vi "Write test data to file polaris.vi"(0 "imei":string="ImeiImeiImeiIme", 1 "Meid":string="MediMeidMeidMe", 4 "SIM ID":string="SimSimSimSimSimSimID", 5 "Mac":string="MacMacMacMac", 7 "phone":string="ImeiImeiImeiIme", 9 "Serial Number":string="MediMeidMeidMe", 11 "error in (no error)":errorcluster, 14 "Style":string="100060") -> (10 "PassFail":string="Fail", 15 "error out":errorcluster)   [LabVIEW 2013]
uses:
  Test Globals/Global 1.vi
  Main Support/Global 2.vi
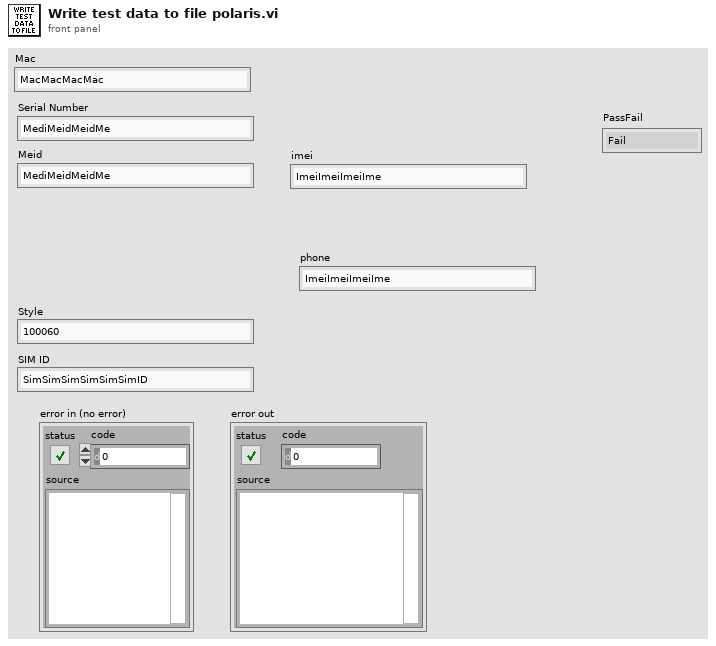
[diagram p1: front panel]
types:
  T1 = enum16{"Query", "Insert", "Select", "Dump Recs", "Get Rec Count", "Get Col Names", "Insert all fields", "Find", "Get last test result", "Get work order qty", "Set work order qty", "Save test report", "Get test report", "Execute query no data", "Select count", "Query and return row 0 col 0"}
  T2 = enum16{"get next serial available and assign", "change status to available", "assign a given serial number"}
  T3 = enum16{"get next serial available and assign", "change status to available"}
  T4 = cluster{"Test folder":string, "Top level":string, "Main":string, "Test report":string, "Work order qty":string, "Work order meid":string, "Work order imei":string, "Master meid imei list":string, "Master test data":string, "ZPL label info":string, "Pictures":string, "Setup info":string, "Work order":string, "Tests folder":string, "Tests steps folder":string, "Config folder":string, "Verizon Upload file":string, "Job data file":string, "Station globals":string, "Post test info":string}
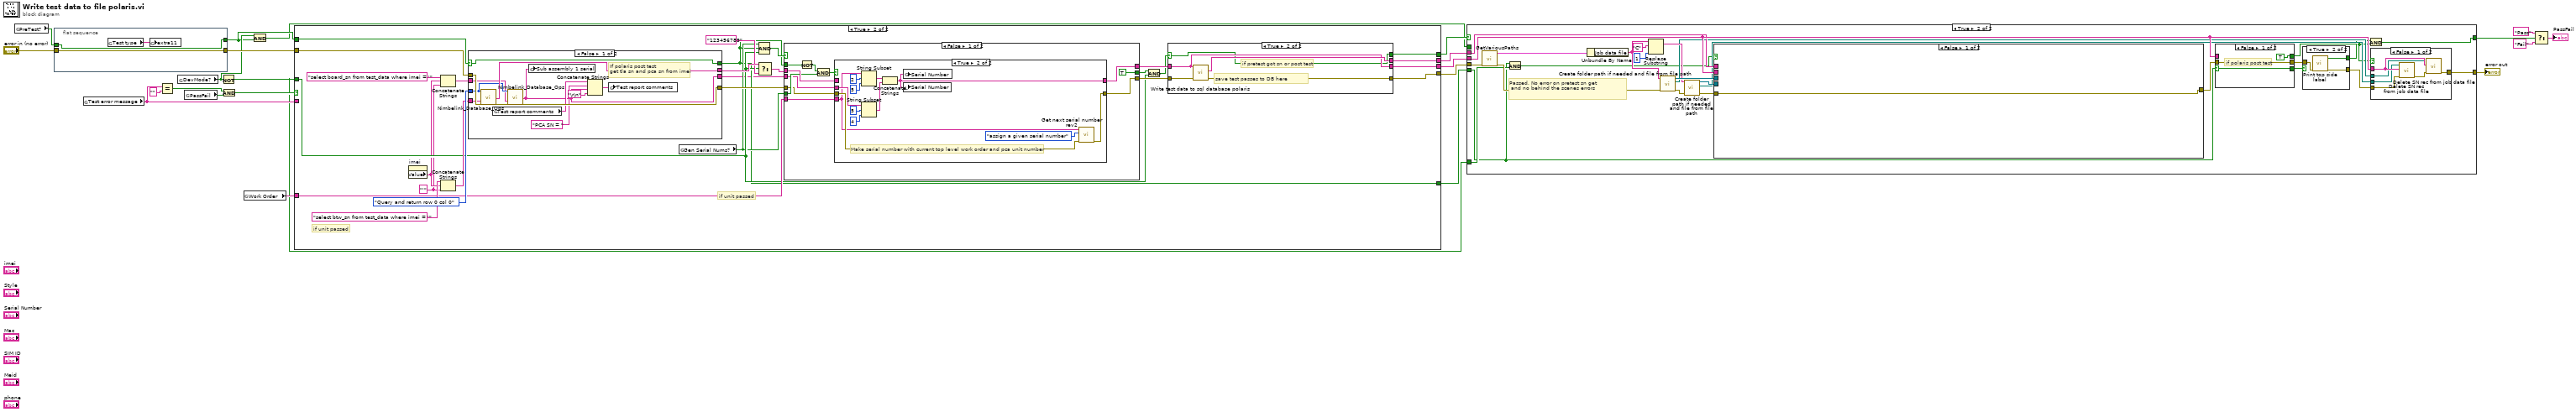
[diagram p0: block diagram]
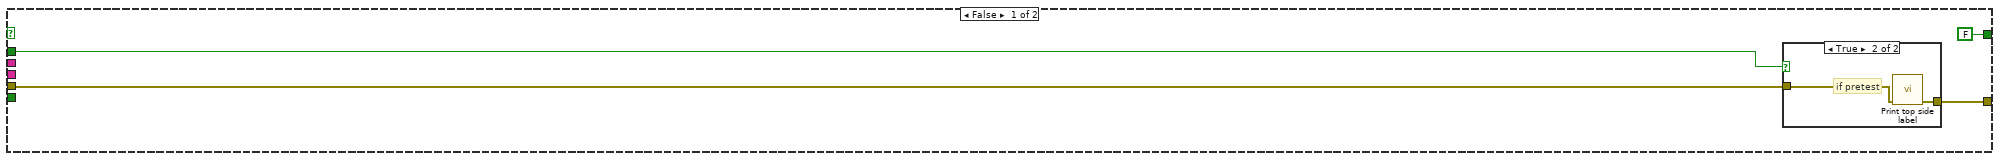
[diagram p2: hidden frame]
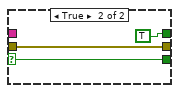
[diagram p4: hidden frame]
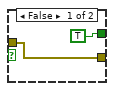
[diagram p5: hidden frame]
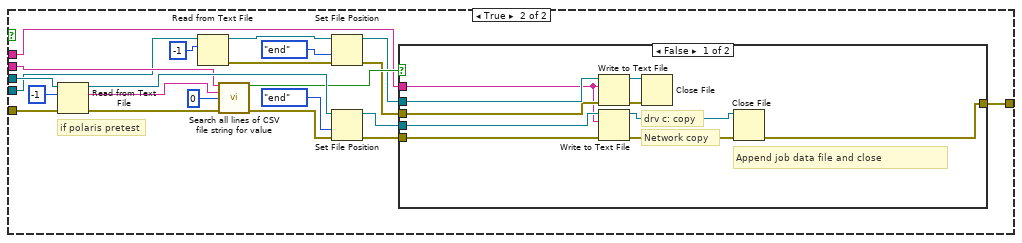
[diagram p7: hidden frame]
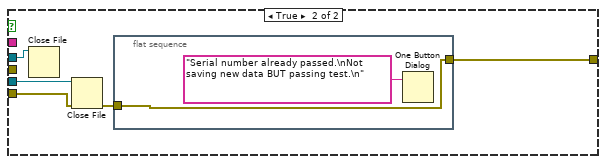
[diagram p8: hidden frame]
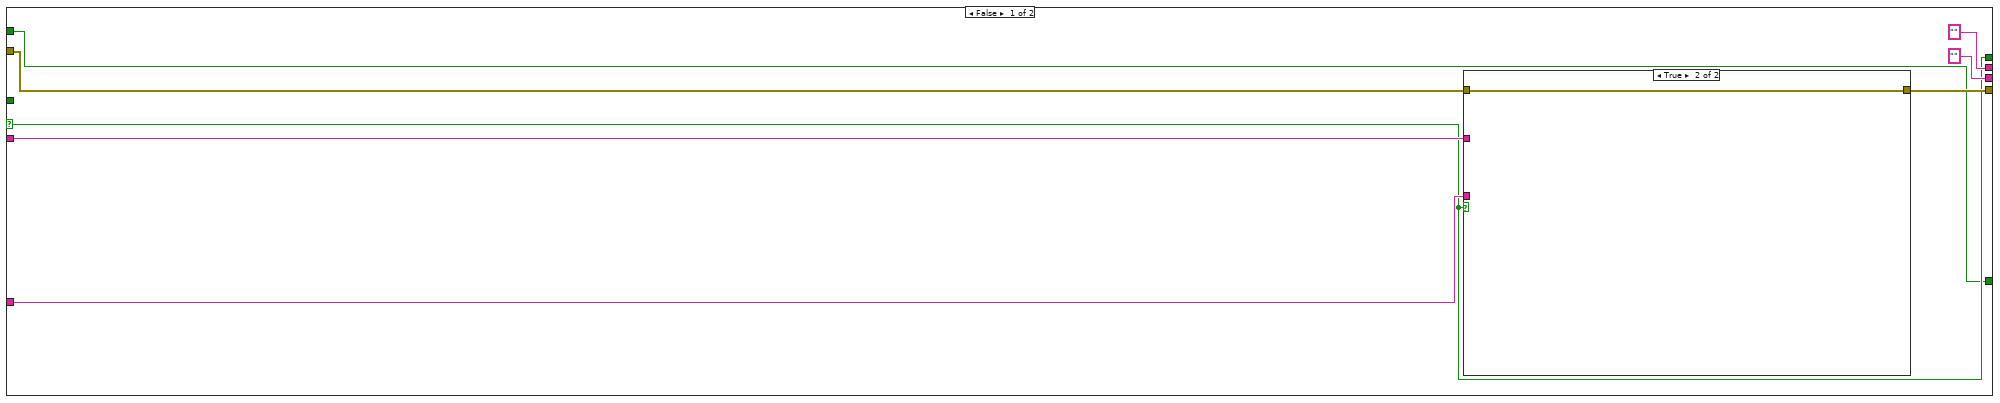
[diagram p9: hidden frame]
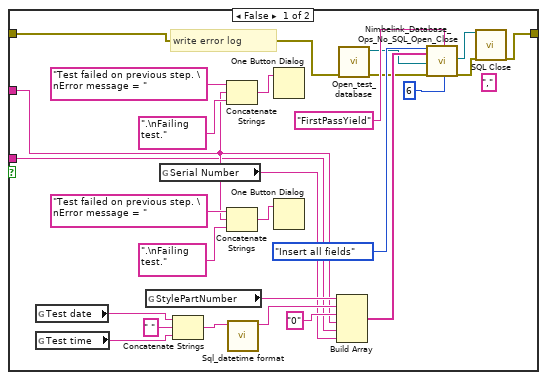
[diagram p10: hidden frame]
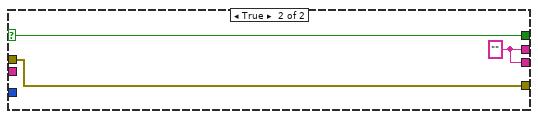
[diagram p11: hidden frame]
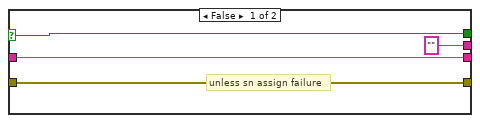
[diagram p12: hidden frame]
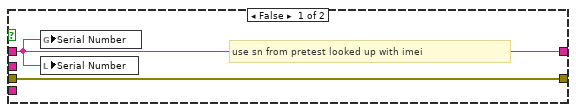
[diagram p13: hidden frame]
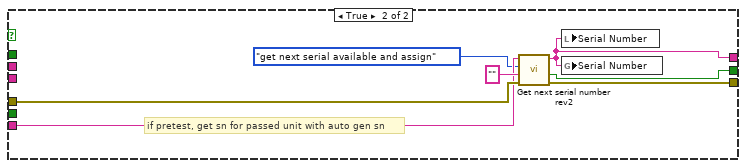
[diagram p14: hidden frame]
diagram:
  n1 = global read "Global 1.vi" "PreTest?"() -> (w7:bool)
  n2 = flat-sequence {
    tunnel: w7 -> [w25]
    tunnel: [w26] -> w9
    tunnel: "error in (no error)" -> [w26]
    tunnel: [w25] -> w2
    frame #0 {
      n3 = global read "Global 1.vi" "Test type"() -> (w24:string)
      n4 = global write "Global 1.vi" "extra11"(w24) -> ()
    }
  }
  n5 = global read "Global 1.vi" "Test error message"() -> (w14:string)
  n6 = Equal?(x=w14, y="") -> (x = y?=w18:bool)
  n7 = global read "Global 1.vi" "DevMode?"() -> (w3:bool)
  n8 = global read "Global 2.vi" "PassFail"() -> (w17:bool)
  n9 = Not(x=w3) -> (.not. x?=w4:bool)
  n10 = And(x=w18, y=w17) -> (x .and. y?=w15:bool)
  n11 = global read "Global 2.vi" "Work Order"() -> (w13:string)
  n12 = And(x=w3, y=w2) -> (x .and. y?=w1:bool)
  n13 = case shown="True" w15 {
    selector: w15 -> [w28 _]
    tunnel: [w30 w85] -> w12
    tunnel: w9 -> [w31 w83]
    tunnel: [w28 w84] -> w5
    tunnel: w14 -> [w34 _]
    tunnel: ["" ("Serial number out") w87] -> w11
    tunnel: ["" ("Test rec csv line") w86] -> w10
    tunnel: w13 -> [w29 w77]
    tunnel: w2 -> [w27 w64]
    tunnel: [w27 w66] -> w6
    tunnel: w4 -> [_ w68]
    frame False {
      n14 = case shown="True" w28 {
        tunnel: w34 -> [w38 _]
        tunnel: w31 -> [w39 w61]
        tunnel: [w37 w61] -> w30
        tunnel: w29 -> [w36 _]
        frame False {
          (unwired) "," ("string")
          # "write error log"
          n15 = global read "Global 2.vi" "Test date"() -> (w48:string)
          n16 = global read "Global 2.vi" "Test time"() -> (w50:string)
          n17 = global read "Global 2.vi" "StylePartNumber"() -> (w51:string)
          n18 = global read "Global 2.vi" "Serial Number"() -> (w35:string)
          n19 = Concatenate Strings(w48, " " ("string"), w50) -> (w47:string)
          n20 = Concatenate Strings("Test failed on previous step. \nError message = " ("string"), w38, ".\nFailing test." ("string")) -> (w60:string)
          n21 = Concatenate Strings("Test failed on previous step. \nError message = " ("string"), w38, ".\nFailing test." ("string")) -> (w57:string)
          n22 = call "Sql_datetime format.vi"("Date time In"=w47) -> ("Sql datetime type 20"=w46:string)  [unwired: 9 in, 1 out]
          n23 = One Button Dialog(message=w60) -> ()  [unwired: 1 in, 1 out]
          n24 = One Button Dialog(message=w57) -> ()  [unwired: 1 in, 1 out]
          n25 = Build Array(w51, w46, "0" ("element"), w38, w36, w35) -> (w44:string[])
          n26 = call "Open_test_database.vi"("error in (no error)"=w39) -> ("error out"=w42:errorcluster, "SQL conn Refnum out"=w43:refnum<k7>)  [unwired: 9 in]
          n27 = call "Nimbelink_Database_Ops_No_SQL_Open_Close.vi"("Operation"=T1."Insert all fields", "Record data"=w44, "Connection In"=w43, "Error in (no error)"=w42, "table name"="FirstPassYield", "Insert fields"=6) -> ("Connection Out"=w40:refnum<k7>, "Error out"=w41:errorcluster)  [unwired: 6 in, 6 out]
          n28 = call "SQL Close.vi"("Connection In"=w40, "Error in (no error)"=w41) -> ("Error out"=w37:errorcluster)  [unwired: 17 in]
        }
        frame True {
        }
      }
    }
    frame True {
      w62 = "'" ("string")
      # "if unit passed"
      # "if unit passed"
      n29 = property on="imei" class="Str"() -> ("Value"=w63:string)  [unwired: 2 in, 2 out]
      n30 = Concatenate Strings("select board_sn from test_data where imei = '" ("SQL Query"), w63, w62) -> (w76:string)
      n31 = Concatenate Strings("select btw_sn from test_data where imei = '" ("SQL Query"), w63, w62) -> (w80:string)
      n32 = case shown="False" w64 {
        selector: w64 -> [w99 w103]
        tunnel: w83 -> [w101 w104]
        tunnel: T1."Query and return row 0 col 0" ("Operation") -> [w96 _]
        tunnel: w80 -> [w100 _]
        tunnel: [w94 w104] -> w75
        tunnel: [w98 w102] -> w73
        tunnel: [w99 w103] -> w66
        tunnel: w76 -> [w95 _]
        tunnel: [w89 w102] -> w65
        frame False {
          # "If polaris post test\nget tla sn and pca sn from imei"
          n33 = call "Nimbelink_Database_Ops.vi"("Operation"=w96, "SQL Query"=w100, "Error in (no error)"=w101) -> ("Find return string"=w98:string, "Error out"=w97:errorcluster)  [unwired: 9 in, 6 out]
          n34 = global read "Global 1.vi" "Test report comments"() -> (w93:string)
          n35 = call "Nimbelink_Database_Ops.vi"("Operation"=w96, "SQL Query"=w95, "Error in (no error)"=w97) -> ("Find return string"=w89:string, "Error out"=w94:errorcluster)  [unwired: 9 in, 6 out]
          n36 = global write "Global 1.vi" "Sub assembly 1 serial"(w89) -> ()
          n37 = Concatenate Strings(w93, "PCA SN = " ("string"), w89, "\r\n") -> (w91:string)
          n38 = global write "Global 1.vi" "Test report comments"(w91) -> ()
        }
        frame True {
          w102 = "" ("Find return string")
        }
      }
      n39 = global read "Global 1.vi" "Gen Serial Nums?"() -> (w67:bool)
      n40 = Select(t=w73, s=w68, f="123456789") -> (s? t:f=w71:string)
      n41 = Compound Arithmetic op=AND(w67, w66, w68) -> (w74:bool)
      n42 = case shown="False" w74 {
        tunnel: w75 -> [w117 w144]
        tunnel: [w116 w142] -> w88
        tunnel: [w118 w139] -> w79
        tunnel: [TRUE ("Got serial number?") w143] -> w70
        tunnel: w77 -> [w114 w141]
        tunnel: w71 -> [w123 _]
        tunnel: w67 -> [w122 _]
        tunnel: w66 -> [w120 _]
        tunnel: w65 -> [w115 _]
        frame False {
          n43 = Not(x=w120) -> (.not. x?=w121:bool)
          n44 = And(x=w121, y=w122) -> (x .and. y?=w119:bool)
          n45 = case shown="True" w119 {
            tunnel: w123 -> [w126 _]
            tunnel: [w126 w134] -> w118
            tunnel: w117 -> [w125 w132]
            tunnel: [w125 w131] -> w116
            tunnel: w115 -> [_ w128]
            tunnel: w114 -> [_ w127]
            frame False {
              # "use sn from pretest looked up with imei"
              n46 = global write "Global 2.vi" "Serial Number"(w126) -> ()
              n47 = local write "Serial Number"(w126) -> ()
            }
            frame True {
              # "Make serial number with current top level work order and pca unit number"
              n48 = String Subset(string=w127, offset (0)=2, length (rest)=5 ("length (rest)")) -> (substring=w136:string)
              n49 = String Subset(string=w128, offset (0)=5, length (rest)=4 ("length (rest)")) -> (substring=w135:string)
              n50 = Concatenate Strings(w136, w135) -> (w134:string)
              n51 = global write "Global 2.vi" "Serial Number"(w134) -> ()
              n52 = local write "Serial Number"(w134) -> ()
              n53 = call "Get next serial number rev2.vi"("Error in (no error)"=w132, "Operation"=T2."assign a given serial number", "Work order (WOXXXXX)"=w127) -> ("Error out"=w131:errorcluster)  [unwired: 6 in, 2 out]
            }
          }
        }
        frame True {
          # "if pretest, get sn for passed unit with auto gen sn"
          n54 = call "Get next serial number rev2.vi"("Error in (no error)"=w144, "Serial number in"="", "Operation"=T3."get next serial available and assign", "Work order (WOXXXXX)"=w141) -> ("Error out"=w142:errorcluster, "OK?"=w143:bool, "Serial Number number out"=w139:string)  [unwired: 5 in]
          n55 = local write "Serial Number"(w139) -> ()
          n56 = global write "Global 2.vi" "Serial Number"(w139) -> ()
        }
      }
      n57 = And(x=w70, y=w68) -> (x .and. y?=w69:bool)
      n58 = case shown="True" w69 {
        selector: w69 -> [w108 w109]
        tunnel: [w107 w111] -> w85
        tunnel: [w108 w109] -> w84
        tunnel: w88 -> [w107 w113]
        tunnel: w79 -> [w106 w110]
        tunnel: [w106 w110] -> w87
        tunnel: ["" ("Test rec csv line") w112] -> w86
        frame False {
          # "unless sn assign failure"
        }
        frame True {
          # "if pretest got sn or post test"
          # "save test passes to DB here"
          n59 = call "Write test data to sql database polaris.vi"("error in (no error)"=w113, "Serial"=w110) -> ("error out"=w111:errorcluster, "Test rec csv line"=w112:string)  [unwired: 4 in, 2 out]
        }
      }
    }
  }
  n60 = case shown="True" w5 {
    tunnel: [FALSE ("Write OK?") w176] -> w20
    tunnel: w12 -> [w148 w175]
    tunnel: [w147 w174] -> w19
    tunnel: w11 -> [_ w173]
    tunnel: w10 -> [_ w170]
    tunnel: w6 -> [_ w153]
    tunnel: w4 -> [_ w155]
    tunnel: w1 -> [w146 _]
    frame False {
      n61 = case shown="True" w146 {
        tunnel: w148 -> [w150 w152]
        tunnel: [w150 w151] -> w147
        frame False {
        }
        frame True {
          # "if pretest"
          n62 = call "Print top side label.vi"("error in (no error)"=w152) -> ("error out"=w151:errorcluster)  [unwired: 7 in, 1 out]
        }
      }
    }
    frame True {
      # "Passed, No error on pretest sn get\n and no behind the scenes errors"
      n63 = call "GetVariousPaths.vi"("error in (no error)"=w175) -> ("error out"=w169:errorcluster, "Built Paths"=w178:T4)  [unwired: 9 in]
      n64 = And(x=w153, y=w155) -> (x .and. y?=w154:bool)
      n65 = Unbundle By Name(w178) -> ("Job data file"=w168:string)
      n66 = Replace Substring(2:1 ("length (len. of substring)"), 4:"C" ("substring (\"\")"), 5:w168) -> (1:w165:string)  [unwired: 1 in, 1 out]
      n67 = call "Create folder path if needed and file from file path.vi"("error in"=w169, "String file path"=w168) -> ("error out"=w166:errorcluster, "file path"=w162:path, "New file refnum"=w167:refnum<file>)  [unwired: 7 in]
      n68 = call "Create folder path if needed and file from file path.vi"("error in"=w166, "String file path"=w165) -> ("error out"=w164:errorcluster, "file path"=w161:path, "New file refnum"=w163:refnum<file>)  [unwired: 7 in]
      n69 = case shown="False" w154 {
        tunnel: w167 -> [_ w213]
        tunnel: w173 -> [_ w209]
        tunnel: w164 -> [w197 w214]
        tunnel: [w197 w206] -> w177
        tunnel: w163 -> [_ w202]
        tunnel: w170 -> [_ w198]
        frame False {
        }
        frame True {
          # "if polaris pretest"
          n70 = Read from Text File(file (use dialog)=w213, count=-1, error in=w214) -> (refnum out=w217:refnum<file>, text=w210:string, error out=w212:errorcluster)  [unwired: 1 in, 1 out]
          n71 = Read from Text File(file (use dialog)=w202, count=-1) -> (refnum out=w205:refnum<file>, error out=w200:errorcluster)  [unwired: 2 in, 2 out]
          n72 = call "Search all lines of CSV file string for value.vi"("Compare value"=w209, "CSV file string"=w210, "CSV field (0-n)"=0, "error in"=w212) -> ("Found value"=w207:bool, "error out"=w211:errorcluster)  [unwired: 10 in]
          n73 = Set File Position(refnum=w205, from (0:start)=enum16{"start", "end", "current"}."end", error in=w200) -> (refnum out=w201:refnum<file>, error out=w199:errorcluster)  [unwired: 1 in]
          n74 = Set File Position(refnum=w217, from (0:start)=enum16{"start", "end", "current"}."end", error in=w211) -> (refnum out=w216:refnum<file>, error out=w215:errorcluster)  [unwired: 1 in]
          n75 = case shown="False" w207 {
            tunnel: w216 -> [w228 w233]
            tunnel: w215 -> [w229 w234]
            tunnel: [w227 w231] -> w206
            tunnel: w201 -> [w222 w230]
            tunnel: w199 -> [w221 _]
            tunnel: w198 -> [w220 _]
            frame False {
              # "Network copy"
              # "drv c: copy"
              # "Append job data file and close"
              n76 = Write to Text File(file (use dialog)=w222, text=w220, error in=w221) -> (refnum out=w224:refnum<file>, error out=w223:errorcluster)  [unwired: 1 in, 1 out]
              n77 = Write to Text File(file (use dialog)=w228, text=w220, error in=w229) -> (refnum out=w225:refnum<file>, error out=w226:errorcluster)  [unwired: 1 in, 1 out]
              n78 = Close File(refnum=w224, error in=w223) -> ()  [unwired: 2 out]
              n79 = Close File(refnum=w225, error in=w226) -> (error out=w227:errorcluster)  [unwired: 1 out]
            }
            frame True {
              n80 = Close File(refnum=w230) -> ()  [unwired: 1 in, 2 out]
              n81 = Close File(refnum=w233, error in=w234) -> (error out=w232:errorcluster)  [unwired: 1 out]
              n82 = flat-sequence {
                tunnel: w232 -> [w236]
                tunnel: [w236] -> w231
                frame #0 {
                  n83 = One Button Dialog(message="Serial number already passed.\nNot saving new data BUT passing test.\n") -> ()  [unwired: 1 in, 1 out]
                }
              }
            }
          }
        }
      }
      n84 = case shown="False" w153 {
        selector: w153 -> [w181 w182]
        tunnel: w177 -> [w180 w184]
        tunnel: w173 -> [_ _]
        tunnel: [w180 w184] -> w160
        tunnel: [TRUE ("Write OK?") TRUE ("Write OK?")] -> w157
        tunnel: [w181 w182] -> w156
        frame False {
          # "if polaris post test"
        }
        frame True {
        }
      }
      n85 = case shown="True" w156 {
        tunnel: w160 -> [w186 w189]
        tunnel: [w186 w188] -> w159
        tunnel: [TRUE ("Print Label OK?") w187] -> w158
        frame False {
        }
        frame True {
          n86 = call "Print top side label.vi"("error in (no error)"=w189) -> ("error out"=w188:errorcluster, "Print Label OK?"=w187:bool)  [unwired: 7 in]
        }
      }
      n87 = And(x=w158, y=w157) -> (x .and. y?=w176:bool)
      n88 = case shown="False" w157 {
        tunnel: w159 -> [w195 w196]
        tunnel: [w192 w196] -> w174
        tunnel: w162 -> [w191 _]
        tunnel: w173 -> [w194 _]
        tunnel: w161 -> [w190 _]
        frame False {
          n89 = call "Delete SN rec from job data file.vi"("error in"=w195, "Serial number"=w194, "file (use dialog)"=w190) -> ("error out"=w193:errorcluster)  [unwired: 8 in]
          n90 = call "Delete SN rec from job data file.vi"("error in"=w193, "Serial number"=w194, "file (use dialog)"=w191) -> ("error out"=w192:errorcluster)  [unwired: 8 in]
        }
        frame True {
        }
      }
    }
  }
  "error out" <- w19
  n91 = Select(t="Pass", s=w20, f="Fail") -> (s? t:f=→"PassFail":string)
